vi "Get Log Directory Path.vi"(8 "error in (no error)":errorcluster, 11 "Plugin Session in":refnum<class "Plugin Session.lvclass">) -> (0 "error out":errorcluster, 2 "Log file directory path":path, 3 "Plugin Session out":refnum<class "Plugin Session.lvclass">)   [LabVIEW 2021, in "Game of Life.lvlib"]
doc: "Gets the directory path for log file"
uses:
  Game of Life.lvlib
  <vilib>/Plug-In SDKs/InstrumentStudio SDK/InstrumentStudioPluginSDK.lvlibp/Plugin Session.lvclass
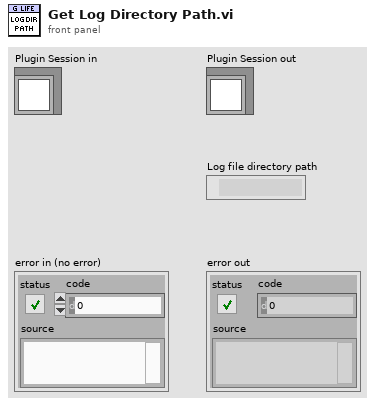
[diagram p1: front panel]
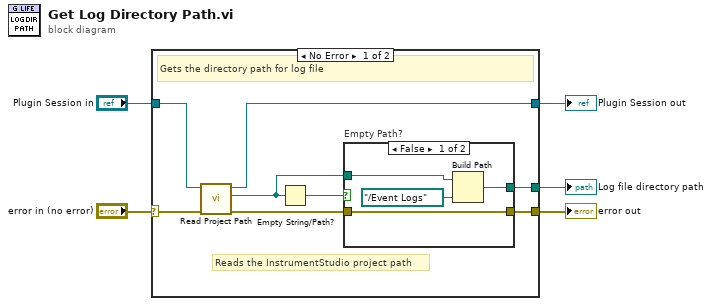
[diagram p0: block diagram]
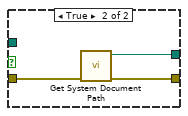
[diagram p2: hidden frame]
diagram:
  n1 = case shown="No Error" "error in (no error)" {
    selector: "error in (no error)" -> [w7 w20]
    tunnel: [w13 w20] -> w5
    tunnel: [w12 _] -> w4
    tunnel: [w8 w21] -> w3
    tunnel: "Plugin Session in" -> [w6 w21]
    frame No Error {
      # "Reads the InstrumentStudio project path"
      # "Gets the directory path for log file"
      n2 = call <vilib>:"Read Project Path.vi"("error in (no error)"=w7, "Session in"=w6) -> ("error out"=w10:errorcluster, "Project Path"=w11:path, "Session out"=w8:refnum<class "Plugin Session.lvclass">)  [unwired: 7 in]
      n3 = Empty String/Path?(string/path=w11) -> (empty?=w9:bool)
      n4 = case "Empty Path?" shown="False" w9 {
        tunnel: w10 -> [w17 w18]
        tunnel: w11 -> [w16 _]
        tunnel: [w14 w19] -> w12
        tunnel: [w17 w18] -> w13
        frame False {
          n5 = Build Path(base path=w16, name or relative path=path "../Event Logs") -> (appended path=w14:path)
        }
        frame True {
          n6 = call "Get System Document Path.vi"() -> ("Public Path"=w19:path)  [unwired: 11 in]
        }
      }
    }
    frame Error {
    }
  }
  "error out" <- w5
  "Log file directory path" <- w4
  "Plugin Session out" <- w3
